vi "19052 Initialize with retry.vi"(7 "Serial Configuration":T1={"Baud Rate"=9600, "Flow Control"=0, "Parity"=0, "Data Bits"=8} {"Baud Rate" items=["300"=300, "600"=600, "1200"=1200, "2400"=2400, "4800"=4800, "9600"=9600, "19200"=19200]; "Flow Control" items=["NONE", "SOFTWARE"]; "Parity" items=["NONE", "ODD", "EVEN"]; "Data Bits" items=["7"=7, "8"=8]}, 8 "error in (no error)":errorcluster, 9 "ID Query (True)":bool=TRUE, 10 "Reset (True)":bool=TRUE, 11 "VISA resource name":refnum<visa-resource-name>) -> (0 "error out":errorcluster, 1 "Message":string, 3 "VISA resource name out":refnum<visa-resource-name>)   [LabVIEW 2025]
uses:
  <vilib>/Utility/error.llb/DialogType.ctl
  <instrlib>/Chroma 19052/Chroma 19052.lvlib
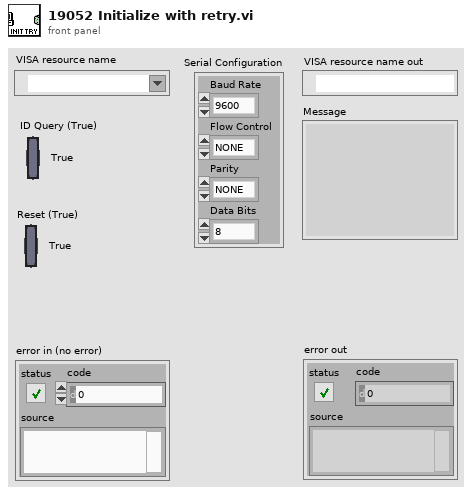
[diagram p1: front panel]
types:
  T1 = cluster{"Baud Rate":u32, "Flow Control":u16, "Parity":u16, "Data Bits":u16}
  T2 = typedef "DialogType.ctl" = u16
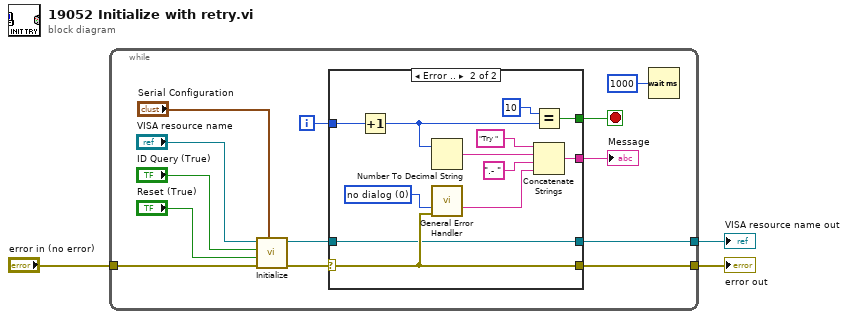
[diagram p0: block diagram]
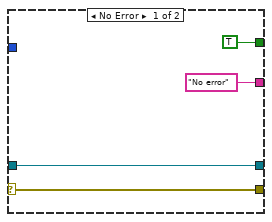
[diagram p2: hidden frame]
diagram:
  n1 = while {
    tunnel: [w11] -> w2
    tunnel: "error in (no error)" -> [w8]
    tunnel: [w7] -> w3
    i -> [w14]
    stop <- w13 stop-if-true
    n2 = call <instrlib>:"Initialize.vi"("Serial Configuration"="Serial Configuration", "error in (no error)"=w8, "Reset (True)"="Reset (True)", "ID Query (True)"="ID Query (True)", "VISA resource name"="VISA resource name") -> ("error out"=w15:errorcluster, "VISA resource name out"=w12:refnum<visa-resource-name>)  [unwired: 5 in]
    n3 = case shown="Error .." w15 {
      selector: w15 -> [w20 w32]
      tunnel: [w20 w32] -> w7
      tunnel: w14 -> [_ w27]
      tunnel: [TRUE w29] -> w13
      tunnel: w12 -> [w18 w31]
      tunnel: [w18 w31] -> w11
      tunnel: ["No error" w22] -> w6
      frame No Error {
      }
      frame Error {
        w30 = T2 0 items=["no dialog", "OK message", "continue or stop message", "OK message + warnings", "continue/stop + warnings"] ("type of dialog (OK msg:1)")
        n4 = Increment(x=w27) -> (x+1=w21:i32)
        n5 = Number To Decimal String(number=w21) -> (decimal integer string=w26:string)  [unwired: 1 in]
        n6 = call <vilib>:"General Error Handler.vi"("type of dialog (OK msg:1)"=w30, "error in (no error)"=w32) -> ("message"=w24:string)  [unwired: 9 in, 4 out]
        n7 = Equal?(x=10 ("y"), y=w21) -> (x = y?=w29:bool)
        n8 = Concatenate Strings("Try " ("string"), w26, ".- " ("string"), w24) -> (w22:string)
      }
    }
    "Message" <- w6
    n9 = Wait (ms)(milliseconds to wait=u32 1000) -> ()  [unwired: 1 out]
  }
  "VISA resource name out" <- w2
  "error out" <- w3
